vi "Write Controlled Devices_HWI.vi"(8 "error in (no error)":errorcluster, 10 "Controlled Devices":T1(array[cluster]), 11 "Arduino in":refnum<class "Arduino.lvclass">) -> (0 "error out":errorcluster, 3 "Arduino out":refnum<class "Arduino.lvclass">)   [LabVIEW 2013, in "Arduino.lvclass"]
uses:
  Arduino.lvclass
  Arduino.lvclass/Arduino.ctl
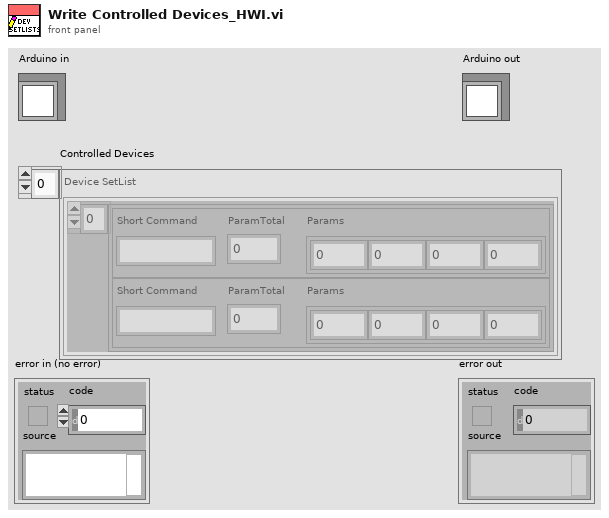
[diagram p1: front panel]
types:
  T1 = cluster{"Array":cluster{"Short Command":string, "ParamTotal":dbl, "Params":dbl[]}[]}[]
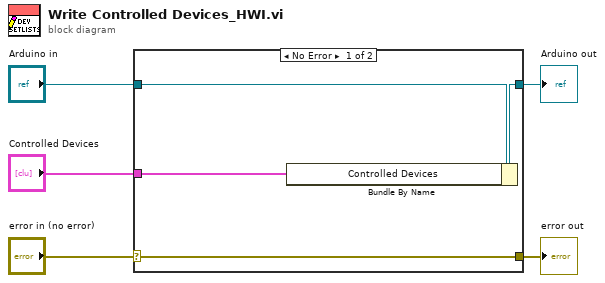
[diagram p0: block diagram]
diagram:
  n1 = case shown="No Error" "error in (no error)" {
    selector: "error in (no error)" -> [w9 w10]
    tunnel: [w9 w10] -> w4
    tunnel: [w7 w11] -> w2
    tunnel: "Arduino in" -> [w8 w11]
    tunnel: "Controlled Devices" -> [w6 _]
    frame No Error {
      n2 = Bundle By Name(cluster=w8, "Controlled Devices"=w6) -> (w7:refnum<class "Arduino.lvclass">)
    }
    frame Error {
    }
  }
  "error out" <- w4
  "Arduino out" <- w2
